vi "Board Control - Configure.vi"() -> ()   [LabVIEW 2020]
uses:
  _controls/port_configuration.ctl
  _controls/port_speed.ctl
  _controls/expert_mode.ctl
  AIM664LV.lvlib
panel:
  in  "Refresh":bool
  in  "Ring":u32(ring) items=["FDX_NO_LINK", "FDX_GOOD_LINK"]
  in  "Stop":bool
  in  "Apply Change to Port":bool
  in  "Port Configuration":enum16{"FDX_SINGLE", "FDX_REDUNDANT"}(ring)
  in  "Expert Mode":enum16{"FDX_EXPERT_MODE", "FDX_DISA_GHOST"}(ring)
  in  "Port Speed":T1(ring)
  in  "ARINC 664 Resources":string[](tree)
  out "NuOfResources":u32
  in  "Server Name":string="local"
  out "Number of Servers":u32=1
  # "ARINC 664 Board Control"
  # "Overview: Queries the boards available in a system and present some properties of those resources.\nRequirement: At least one AIM ARINC-664 board with installed AIM ARINC 664 BSP.\nRestrictions: None.\nInstruction:\n1. Run the VI.\n2. Verify the resources available. If no error is presented, you will see all of the resources in the Resources."
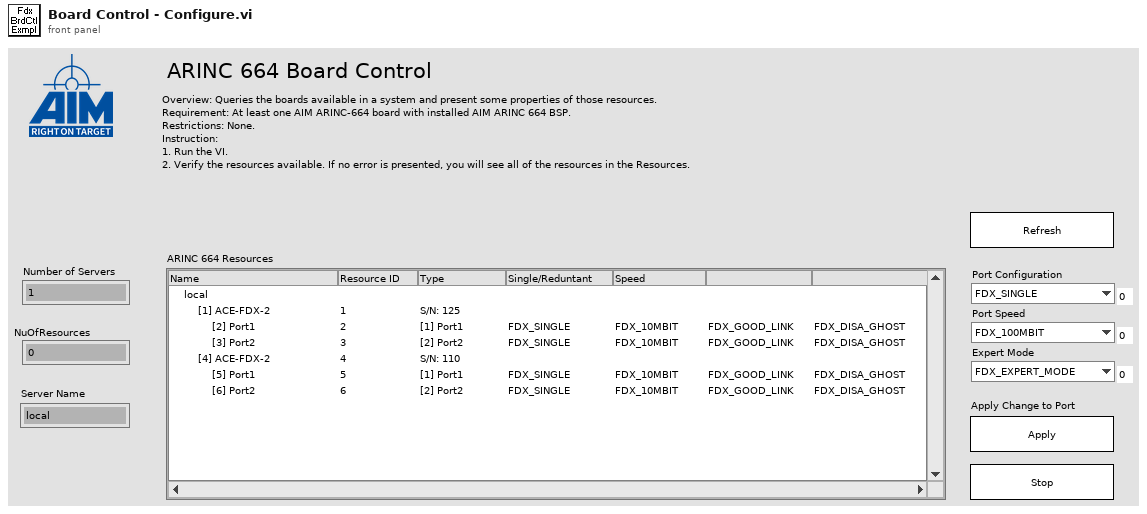
[diagram p1: front panel]
types:
  T1 = enum16{"FDX_100MBIT", "FDX_10MBIT", "FDX_AUTO_100MBIT", "FDX_AUTO_10MBIT", "FDX_1000MBIT"}
  T2 = cluster{"BoardName":string, "BoardSerialNo":u32, "BoardNumOf\nEthernetPorts":u32, "BoardClients":u32, "BoardGlobal\nMemSize":u32, "BoardShared\nMemSize":u32, "BoardStructId":u32, "PortName":string, "PortMode":u32, "PortNo":u32, "PortBoard\nResourceID":u32, "PortStructId":u32}
  T3 = typedef "AIM664LV.lvlib/port_configuration.ctl" = u32
  T4 = typedef "AIM664LV.lvlib/port_speed.ctl" = u32
  T5 = typedef "AIM664LV.lvlib/port_condition.ctl" = u32
  T6 = typedef "AIM664LV.lvlib/expert_mode.ctl" = u32
  T7 = cluster{"PortConfig":T3[], "PortSpeed":T4[], "PortUsed":u32[], "PortGoodLink":T5[], "ExpertMode":T6[], "GlobalMemFree":u32, "SharedMemFree":u32, "RxVeriMode":u32}
  T8 = cluster{"Left Cell String":string, "Child Text":string[], "Child Tag":string, "Item Indent":i32, "Child Only?":bool, "Glyph Index":i32}
  T9 = cluster{"Left Cell String":string, "Child Text":string[], "Child Tag":string, "Item Indent":i32, "Child Only?":bool, "Glyph Index":i32}[]
  T10 = cluster{"Control":u32, "Port1ConfigIn":T3, "Port2ConfigIn":T3, "Port3ConfigIn":T3, "Port4ConfigIn":T3, "Port1SpeedIn":T4, "Port2SpeedIn":T4, "Port3SpeedIn":T4, "Port4SpeedIn":T4, "Expert1Mode":T6, "Expert2Mode":T6, "Expert3Mode":T6, "Expert4Mode":T6, "RxVeriModeIn":u32, "RxVeriData1":u32, "RxVeriData2":u32, "RxVeriData3":u32, "RxVeriData4":u32, "RxVeriData5":u32, "RxVeriData6":u32, "RxVeriData7":u32, "RxVeriData8":u32, "RxVeriMask1":u32, "RxVeriMask2":u32, "RxVeriMask3":u32, "RxVeriMask4":u32, "RxVeriMask5":u32, "RxVeriMask6":u32, "RxVeriMask7":u32, "RxVeriMask8":u32}
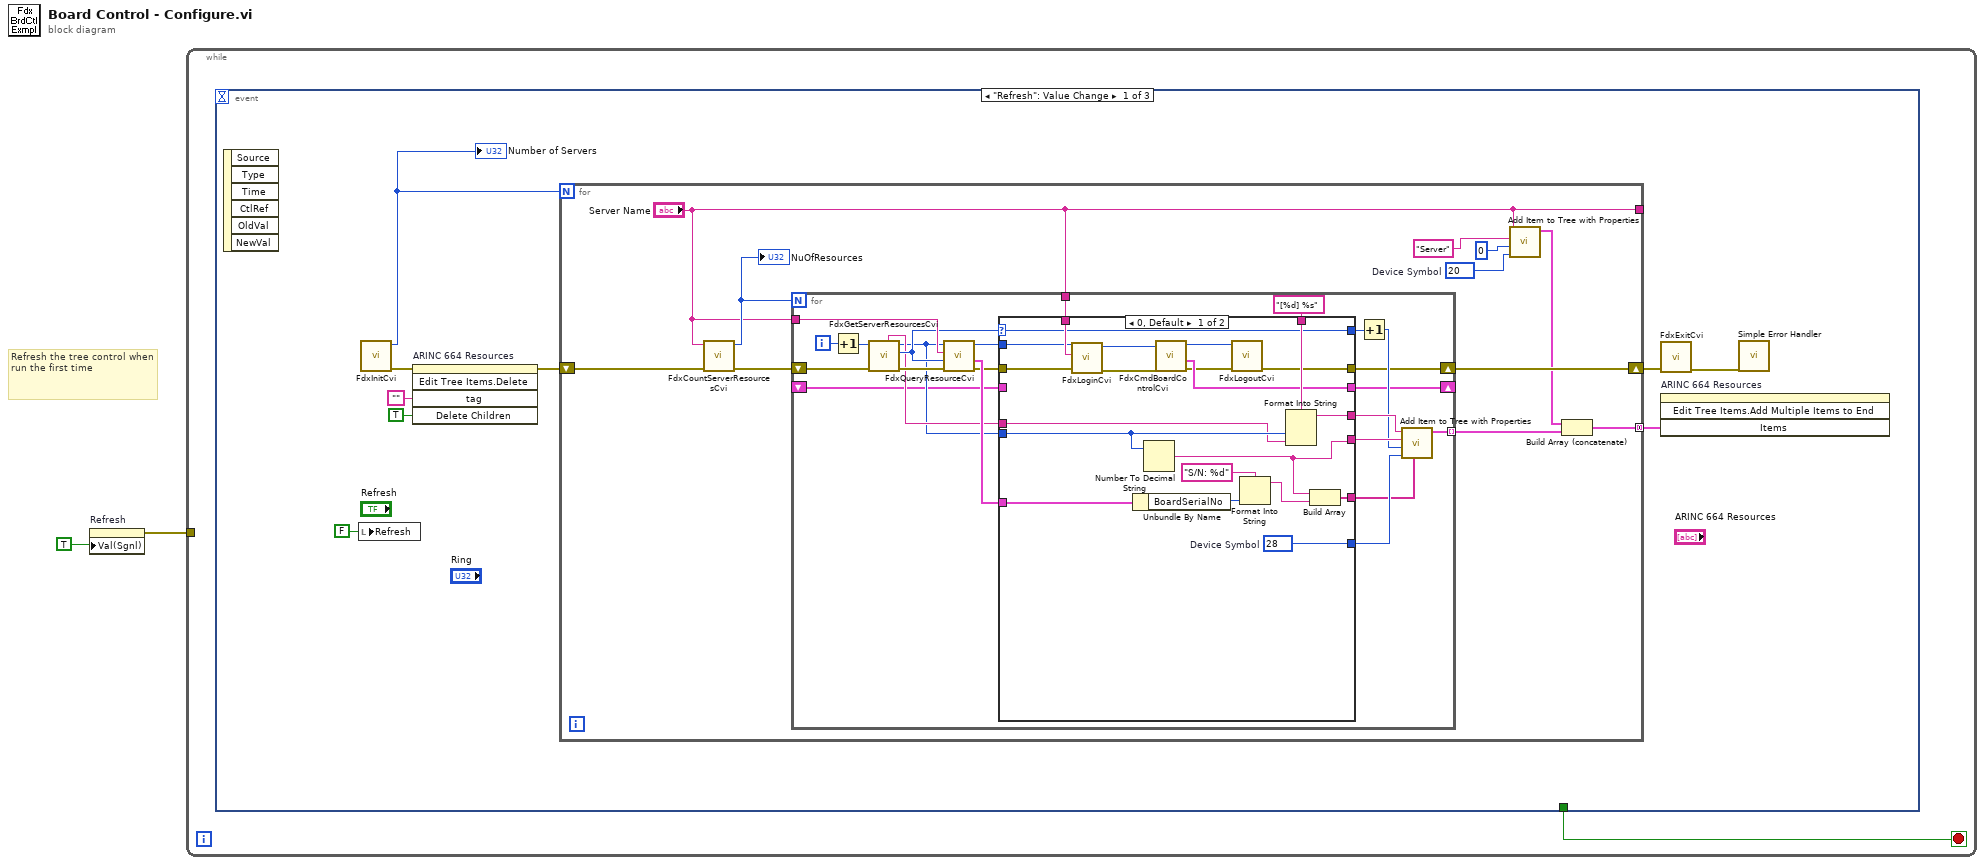
[diagram p0: block diagram]
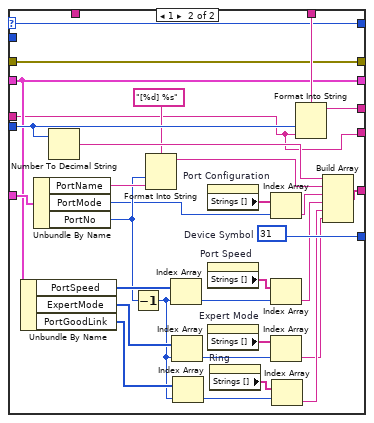
[diagram p2: hidden frame]
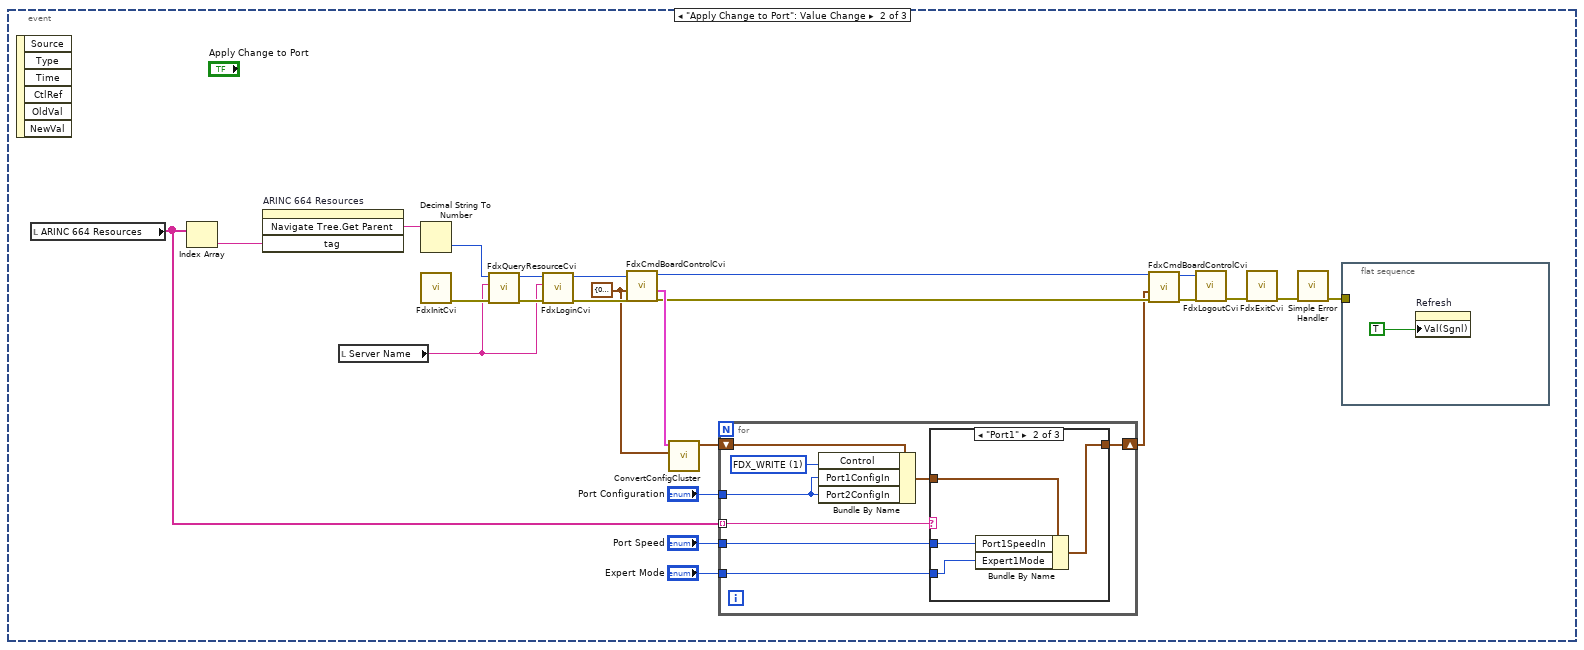
[diagram p3: hidden frame]
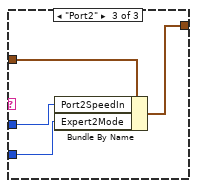
[diagram p5: hidden frame]
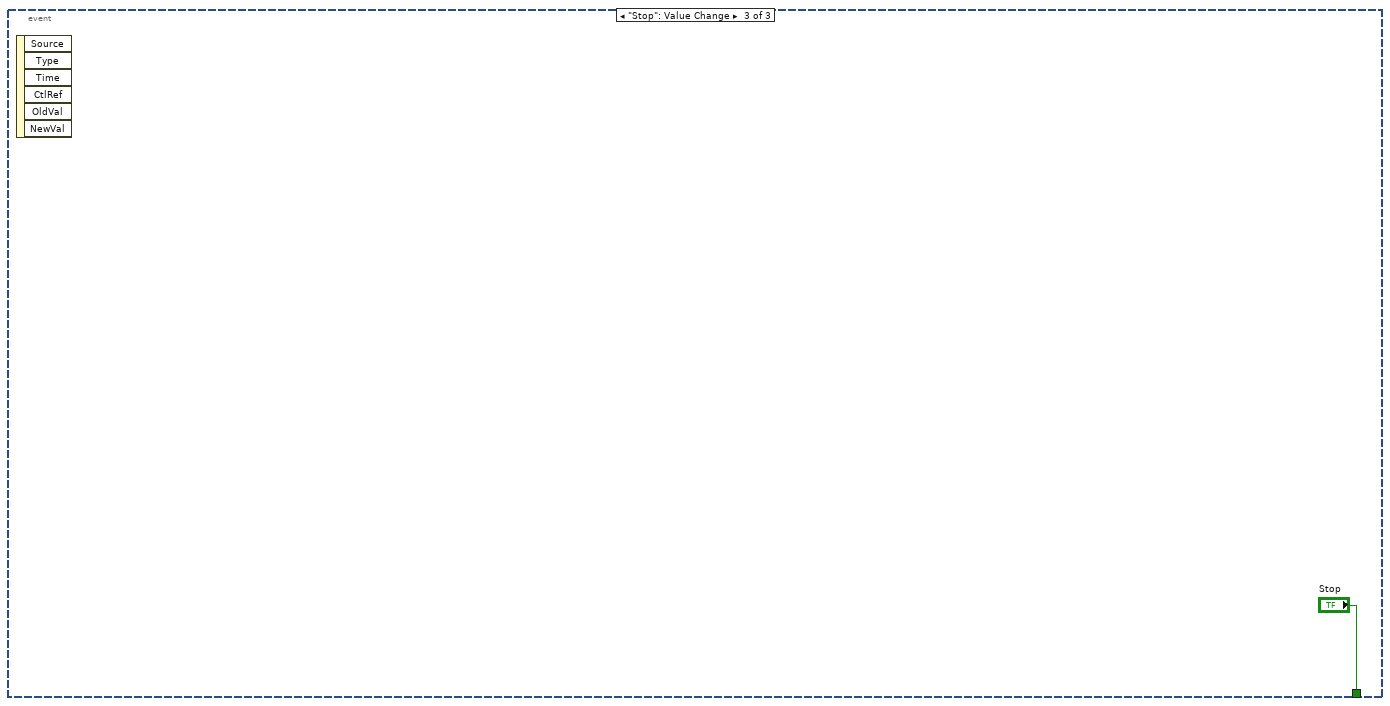
[diagram p6: hidden frame]
diagram:
  # "Refresh the tree control when run the first time"
  n1 = property on="Refresh" class="Bool (strict)"("Val(Sgnl)"=TRUE) -> (error out=w2:errorcluster)  [unwired: 2 in, 1 out]
  n2 = while {
    tunnel: w2 -> [_]
    stop <- w3 stop-if-true
    n3 = event shown="[0] \"Refresh\": Value Change" {
      selector: _ -> [_ _ _]
      dyn-events: _ -> [_ _ _]
      timeout: _ -> [_ _ _]
      tunnel: [_ _ "Stop"] -> w3
      event "Refresh": Value Change {
        n4 = event-data() -> ()  [unwired: 1 in, 6 out]
        n5 = local write "Refresh"(FALSE ("Refresh")) -> ()
        n6 = call "FdxInitCvi.vi"() -> ("error out"=w10:errorcluster, "Number of Servers"=w12:u32)  [unwired: 10 in]
        "Number of Servers" <- w12
        n7 = invoke on="ARINC 664 Resources" class="Tree (strict)" method="Edit Tree Items.Delete"(error in=w10, "tag"="", "Delete Children"=TRUE ("Delete Children?")) -> (error out=w9:errorcluster)  [unwired: 2 in, 4 out]
        n8 = for {
          N: w12 -> [_]
          shift-right: [w21] -> w6
          shift-left: w9 -> [w23]
          tunnel: [w18] -> w11 mode=concatenating
          tunnel: ["Server Name"] -> _
          w16 = 20  # Device Symbol
          n9 = call "FdxCountServerResourcesCvi.vi"("error in"=w23, "SrvName (local)"="Server Name") -> ("error out"=w22:errorcluster, "Number of Resources"=w20:u32)  [unwired: 8 in]
          "NuOfResources" <- w20
          n10 = for {
            N: w20 -> [_]
            shift-right: [w28] -> w21
            shift-left: w22 -> [w46]
            tunnel: [w43] -> w19 mode=indexing
            tunnel: "Server Name" -> [w39]
            shift-right: [w27] -> _
            shift-left: _ -> [w26]
            tunnel: "Server Name" -> [w25]
            i -> [w44]
            n11 = Increment(x=w44) -> (x+1=w41:i32)
            n12 = call "FdxGetServerResourcesCvi.vi"("error in"=w46, "ServerRElement"=w41) -> ("error out"=w40:errorcluster, "ResourceType"=w38:u32, "Resource ID"=w35:u32, "Resource Info"=w36:string)  [unwired: 4 in, 2 out]
            n13 = call "FdxQueryResourceCvi.vi"("error in"=w40, "ResourceType"=w38, "SrvName"=w39, "ResourceID"=w35) -> ("error out"=w30:errorcluster, "ResourceInfo"=w37:T2, "ResourceID out"=w29:u32)  [unwired: 5 in]
            n14 = case shown="0, Default" w38 {
              selector: w38 -> [w49 w75]
              tunnel: [w67 w98] -> w45
              tunnel: [w47 w74] -> w42
              tunnel: w37 -> [w65 w96]
              tunnel: w36 -> [w48 w74]
              tunnel: w35 -> [w59 w93]
              tunnel: [w60 w94] -> w34
              tunnel: "[%d] %s" ("format string") -> [w66 w97]
              tunnel: [w64 w95] -> w32
              tunnel: w30 -> [w57 w88]
              tunnel: w29 -> [w54 _]
              tunnel: [w51 w88] -> w28
              tunnel: [w58 w86] -> w27
              tunnel: w26 -> [_ w86]
              tunnel: w25 -> [w55 _]
              tunnel: [w49 w75] -> w24
              frame 0, Default {
                w67 = 28  # Device Symbol
                n15 = call "FdxLoginCvi.vi"("error in"=w57, "SrvName"=w55, "ResourceID"=w54) -> ("error out"=w56:errorcluster, "InstrumentHandle"=w53:u32)  [unwired: 7 in]
                n16 = Unbundle By Name(w65) -> ("BoardSerialNo"=w63:u32)
                n17 = Number To Decimal String(number=w59) -> (decimal integer string=w47:string)  [unwired: 1 in]
                n18 = call "FdxCmdBoardControlCvi.vi"("error in"=w56, "InstrumentHandle_board in"=w53) -> ("error out"=w52:errorcluster, "Board Control Out"=w58:T7, "InstrumentHandle_board out"=w50:u32)  [unwired: 7 in]
                n19 = call "FdxLogoutCvi.vi"("error in"=w52, "InstrumentHandle"=w50) -> ("error out"=w51:errorcluster)  [unwired: 9 in]
                n20 = Format Into String(format string="S/N: %d", w63) -> (resulting string=w62:string)  [unwired: 2 in, 1 out]
                n21 = Format Into String(format string=w66, w59, w48) -> (resulting string=w60:string)  [unwired: 2 in, 1 out]
                n22 = Build Array(w47, w62) -> (w64:string[])
              }
              frame 1 {
                w98 = 31  # Device Symbol
                n23 = Unbundle By Name(w86) -> ("PortSpeed"=w87:T4[], "ExpertMode"=w81:T6[], "PortGoodLink"=w73:T5[])
                n24 = Unbundle By Name(w96) -> ("PortName"=w90:string, "PortMode"=w76:u32, "PortNo"=w79:u32)
                n25 = Number To Decimal String(number=w93) -> (decimal integer string=w92:string)  [unwired: 1 in]
                n26 = Decrement(x=w79) -> (x-1=w72:u32)
                n27 = Format Into String(format string="[%d] %s", w79, w90) -> (resulting string=w91:string)  [unwired: 2 in, 1 out]
                n28 = Index Array(array=w87, index=w72) -> (element=w85:T4)
                n29 = Index Array(array=w81, index=w72) -> (element=w82:T6)
                n30 = Index Array(array=w73, index=w72) -> (element=w70:T5)
                n31 = property on="Port Configuration" class="Enum (strict)"() -> ("Strings []"=w78:string[])  [unwired: 2 in, 2 out]
                n32 = property on="Port Speed" class="Enum (strict)"() -> ("Strings []"=w84:string[])  [unwired: 2 in, 2 out]
                n33 = property on="Expert Mode" class="Enum (strict)"() -> ("Strings []"=w80:string[])  [unwired: 2 in, 2 out]
                n34 = property on="Ring" class="Ring (strict)"() -> ("Strings []"=w71:string[])  [unwired: 2 in, 2 out]
                n35 = Index Array(array=w78, index=w76) -> (element=w77:string)
                n36 = Index Array(array=w84, index=w85) -> (element=w83:string)
                n37 = Index Array(array=w80, index=w82) -> (element=w68:string)
                n38 = Index Array(array=w71, index=w70) -> (element=w69:string)
                n39 = Format Into String(format string=w97, w93, w74) -> (resulting string=w94:string)  [unwired: 2 in, 1 out]
                n40 = Build Array(w92, w91, w77, w83, w69, w68) -> (w95:string[])
              }
            }
            n41 = Increment(x=w24) -> (x+1=w31:u32)
            n42 = call "Add Item to Tree with Properties.vi"("Child Text"=w32, "Glyph Index"=w45, "Item indent"=w31, "Child Tag"=w42, "Left Cell String"=w34) -> ("Item"=w43:T8)  [unwired: 6 in]
          }
          n43 = call "Add Item to Tree with Properties.vi"("Glyph Index"=w16, "Item indent"=0, "Child Tag"="Server", "Left Cell String"="Server Name") -> ("Item"=w17:T8)  [unwired: 7 in]
          n44 = Build Array (concatenate)(w17, w19) -> (w18:T9)
        }
        n45 = call "FdxExitCvi.vi"("error in"=w6) -> ("error out"=w5:errorcluster)  [unwired: 10 in]
        n46 = invoke on="ARINC 664 Resources" class="Tree (strict)" method="Edit Tree Items.Add Multiple Items to End"("Items"=w11) -> ()  [unwired: 3 in, 4 out]
        n47 = call <vilib>:"Simple Error Handler.vi"("error in (no error)"=w5) -> ()  [unwired: 4 in, 5 out]
      }
      event "Apply Change to Port": Value Change {
        w99 = T10 {"Control"=0, "Port1ConfigIn"=0, "Port2ConfigIn"=0, "Port3ConfigIn"=0, "Port4ConfigIn"=0, "Port1SpeedIn"=0, "Port2SpeedIn"=0, "Port3SpeedIn"=0, "Port4SpeedIn"=0, "Expert1Mode"=0, "Expert2Mode"=0, "Expert3Mode"=0, "Expert4Mode"=0, "RxVeriModeIn"=0, "RxVeriData1"=0, "RxVeriData2"=0, "RxVeriData3"=0, "RxVeriData4"=0, "RxVeriData5"=0, "RxVeriData6"=0, "RxVeriData7"=0, "RxVeriData8"=0, "RxVeriMask1"=0, "RxVeriMask2"=0, "RxVeriMask3"=0, "RxVeriMask4"=0, "RxVeriMask5"=0, "RxVeriMask6"=0, "RxVeriMask7"=0, "RxVeriMask8"=0} ("BoardControlIn (read)")
        n48 = event-data() -> ()  [unwired: 1 in, 6 out]
        n49 = local read "ARINC 664 Resources"() -> (w104:string[])
        n50 = Index Array(array=w104) -> (element=w113:string)  [unwired: 1 in]
        n51 = invoke on="ARINC 664 Resources" class="Tree (strict)" method="Navigate Tree.Get Parent"("tag"=w113) -> ("Navigate Tree:Get Parent"=w117:string)  [unwired: 3 in, 3 out]
        n52 = local read "Server Name"() -> (w115:string)
        n53 = Decimal String To Number(string=w117) -> (number=w119:i32)  [unwired: 2 in, 1 out]
        n54 = call "FdxInitCvi.vi"() -> ("error out"=w122:errorcluster)  [unwired: 10 in, 1 out]
        n55 = call "FdxQueryResourceCvi.vi"("error in"=w122, "SrvName"=w115, "ResourceID"=w119) -> ("error out"=w121:errorcluster, "ResourceID out"=w118:u32)  [unwired: 6 in, 1 out]
        n56 = call "FdxLoginCvi.vi"("error in"=w121, "SrvName"=w115, "ResourceID"=w118) -> ("error out"=w111:errorcluster, "InstrumentHandle"=w112:u32)  [unwired: 7 in]
        n57 = call "FdxCmdBoardControlCvi.vi"("error in"=w111, "BoardControlIn (read)"=w99, "InstrumentHandle_board in"=w112) -> ("error out"=w105:errorcluster, "Board Control Out"=w110:T7, "InstrumentHandle_board out"=w108:u32)  [unwired: 6 in]
        n58 = call "ConvertConfigCluster.vi"("Original Board Control In"=w99, "Board Control Output"=w110) -> ("Adjusted Board Control Input"=w109:T10)  [unwired: 9 in]
        n59 = for {
          tunnel: w104 -> [w128] mode=indexing
          shift-right: [w126] -> w103
          shift-left: w109 -> [w127]
          tunnel: "Expert Mode" -> [w125]
          tunnel: "Port Speed" -> [w124]
          tunnel: "Port Configuration" -> [w123]
          w130 = u32 1 items=["FDX_READ", "FDX_WRITE"] ("Control")
          n60 = Bundle By Name(cluster=w127, "Control"=w130, "Port1ConfigIn"=w123, "Port2ConfigIn"=w123) -> (w129:T10)
          n61 = case shown="\"Port1\"" w128 {
            tunnel: w129 -> [w131 w135 w139]
            tunnel: w124 -> [_ w134 w138]
            tunnel: w125 -> [_ w133 w137]
            tunnel: [w131 w132 w136] -> w126
            frame Default {
            }
            frame "Port1" {
              n62 = Bundle By Name(cluster=w135, "Port1SpeedIn"=w134, "Expert1Mode"=w133) -> (w132:T10)
            }
            frame "Port2" {
              n63 = Bundle By Name(cluster=w139, "Port2SpeedIn"=w138, "Expert2Mode"=w137) -> (w136:T10)
            }
          }
        }
        n64 = call "FdxCmdBoardControlCvi.vi"("error in"=w105, "BoardControlIn (read)"=w103, "InstrumentHandle_board in"=w108) -> ("error out"=w106:errorcluster, "InstrumentHandle_board out"=w107:u32)  [unwired: 6 in, 1 out]
        n65 = call "FdxLogoutCvi.vi"("error in"=w106, "InstrumentHandle"=w107) -> ("error out"=w120:errorcluster)  [unwired: 9 in]
        n66 = call "FdxExitCvi.vi"("error in"=w120) -> ("error out"=w116:errorcluster)  [unwired: 10 in]
        n67 = call <vilib>:"Simple Error Handler.vi"("error in (no error)"=w116) -> ("error out"=w114:errorcluster)  [unwired: 4 in, 4 out]
        n68 = flat-sequence {
          tunnel: w114 -> [_]
          frame #0 {
            n69 = property on="Refresh" class="Bool (strict)"("Val(Sgnl)"=TRUE ("Value (Signaling)")) -> ()  [unwired: 2 in, 2 out]
          }
        }
      }
      event "Stop": Value Change {
        n70 = event-data() -> ()  [unwired: 1 in, 6 out]
      }
    }
  }
